vi "Main.vi"(11 "Error in":errorcluster) -> (15 "Error out":errorcluster)   [LabVIEW 2020, in "PSRR Monitor.lvlib"]
uses:
  PSRR Monitor.lvlib
  Typedefs/Queue operations.ctl
  Typedefs/Data Cluster.ctl
  Typedefs/Variant cluster.ctl
  Typedefs/User LV2 operations.ctl
  Typedefs/User LV2 data.ctl
  <vilib>/Utility/config.llb/Read Key (I32).vi
  <vilib>/Utility/config.llb/Read Key (Boolean).vi
  SubVI/Error log.vi
  <vilib>/Utility/config.llb/Write Key (I32).vi
  <vilib>/Utility/config.llb/Write Key (Boolean).vi
  <vilib>/Utility/config.llb/NI_LVConfig.lvlib
panel:
  out "Obtained PSRR":i32(graph)
  in  "Error Log":bool
  in  "Exit":bool
  out "Description":string
  out "Time":string
  out "Type":string
  out "Error Code":i32
  out "Last Read PSRR (dB)":i32
  in  "Wait Time(sec)":i32 min=2 step=1
  out "Error?":bool
  # "PSRR MONITOR"
  # "Power Supply Rejection Ratio"
  # "Last Error Details"
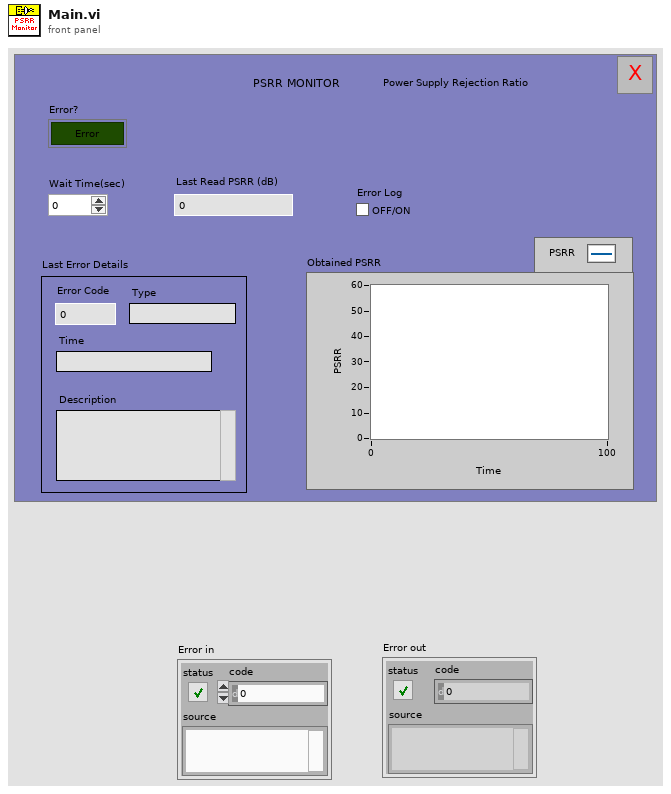
[diagram p1: front panel]
types:
  T1 = typedef "User LV2 operations.ctl" = enum16{"Destroy", "Get ref", "Generate", "Create"}
  T2 = typedef "PSRR Monitor.lvlib/Variant cluster.ctl" = cluster{"State":string, "Data":variant}
  T3 = typedef "PSRR Monitor.lvlib/Queue operations.ctl" = enum16{"Create", "Enqueue", "Enstack", "Dequeue", "Flush", "Release "}
  T4 = typedef "PSRR Monitor.lvlib/Data Cluster.ctl" = cluster{"Error?":bool, "Exit":bool, "Error log":bool, "Type":string, "Time":string, "Description":string, "Wait Time":i32, "Last Read PSRR":i32, "Error code":i32, "Obtained PSRR":i32, "Start/Stop Timer":bool, "Start time":dbl, "Path":path, "Passive count":dbl, "Other error count":dbl}
  T5 = typedef "User LV2 data.ctl" = cluster{"Exit":bool}
  T6 = typedef "NI_LVConfig.lvlib/Config Data RefNum.ctl" = refnum<k1>
  T7 = enum32{"Bad", "Idle", "Run top level", "Running"}
  T8 = typedef "PSRR Monitor.lvlib/Error Details.ctl" = cluster{"Error Code":i32, "Error Type":string, "Time":string, "Description":string, "PSRR":i32}
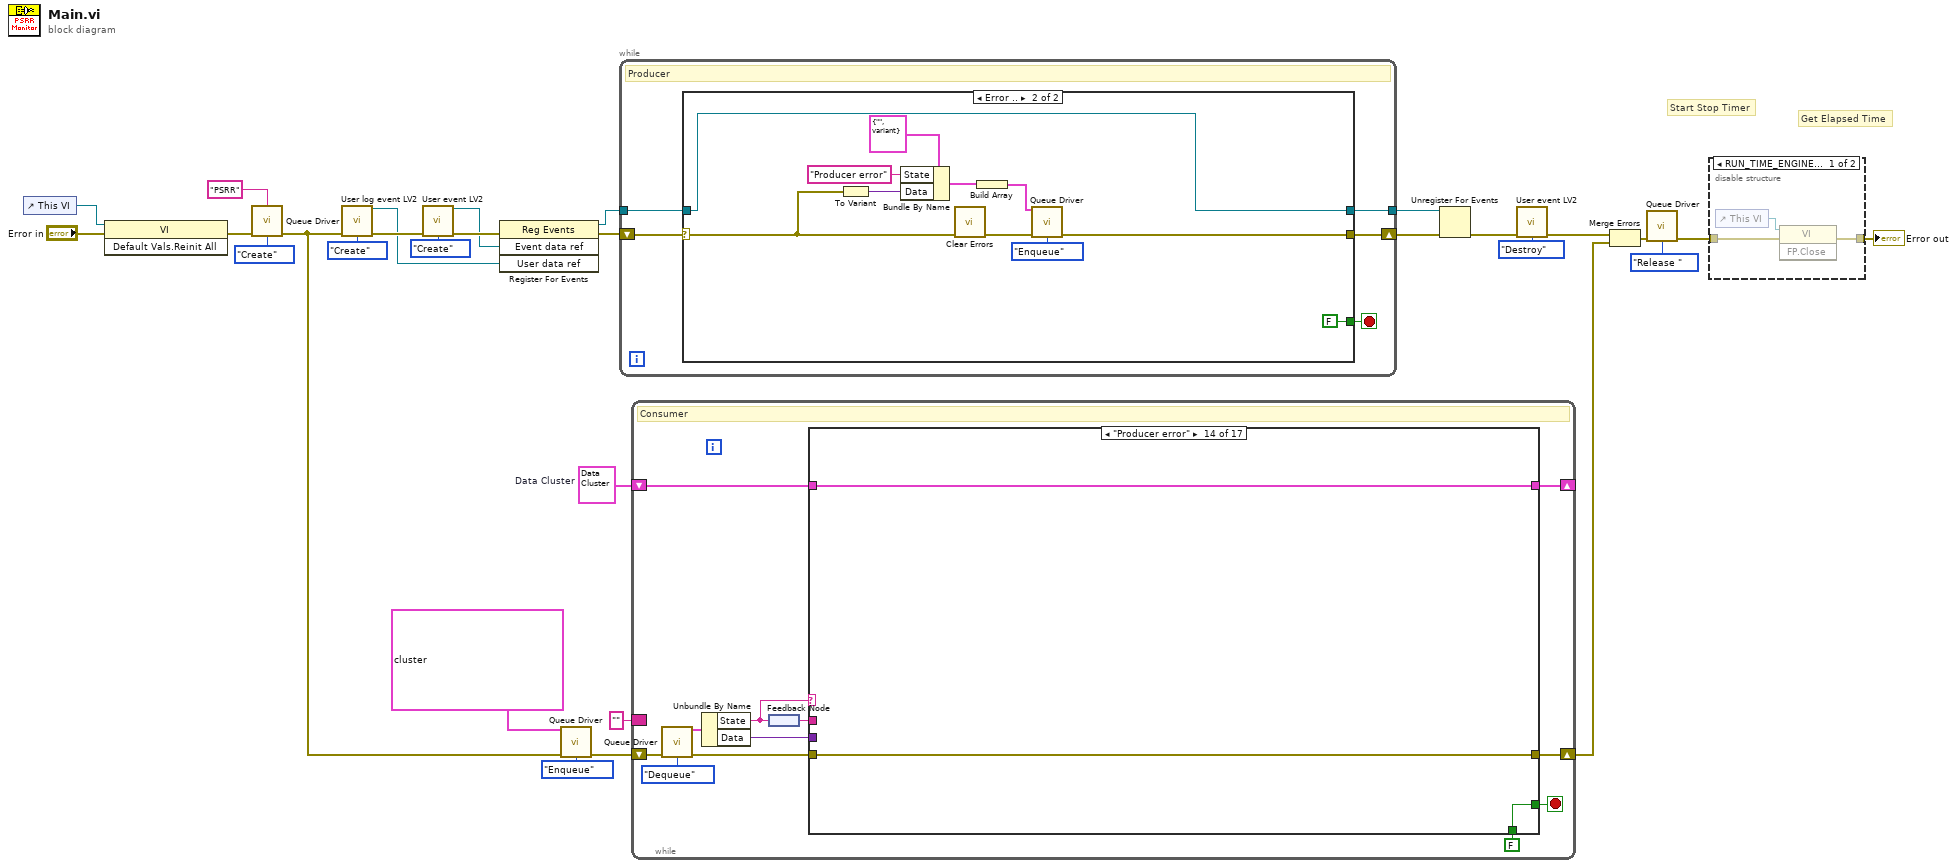
[diagram p0: block diagram]
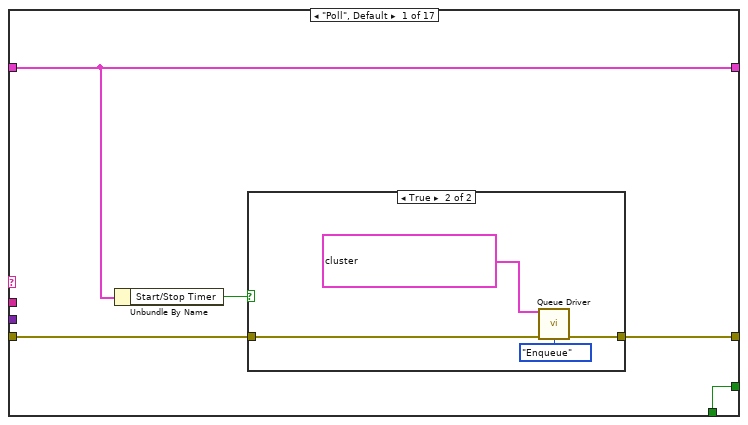
[diagram p3: hidden frame]
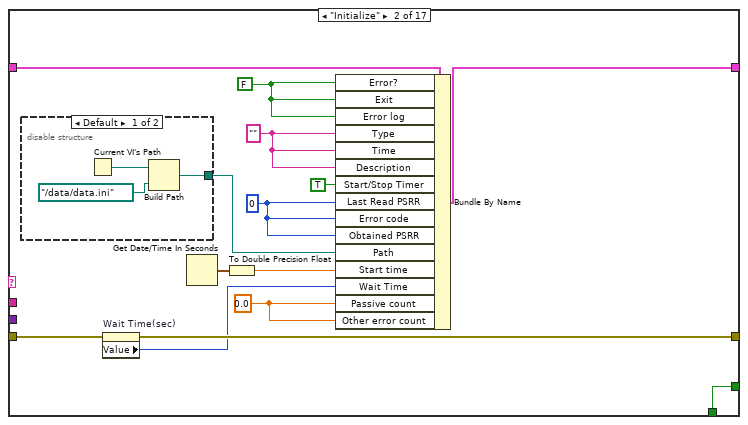
[diagram p5: hidden frame]
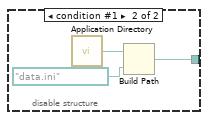
[diagram p6: hidden frame]
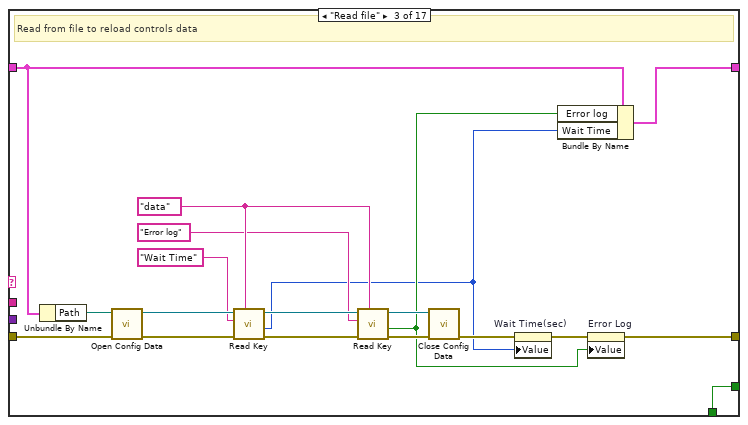
[diagram p7: hidden frame]
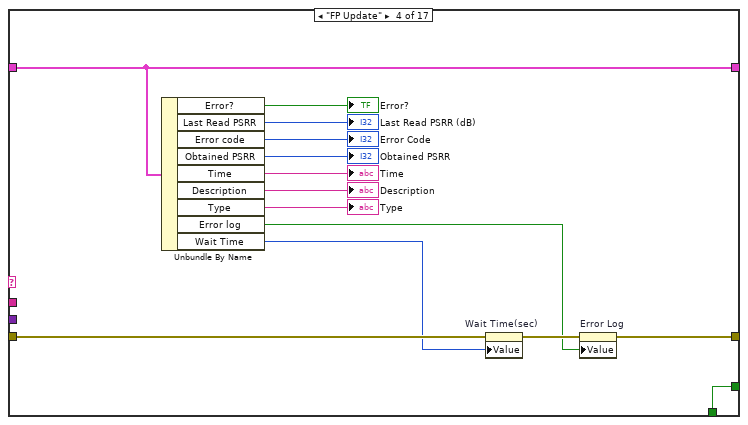
[diagram p8: hidden frame]
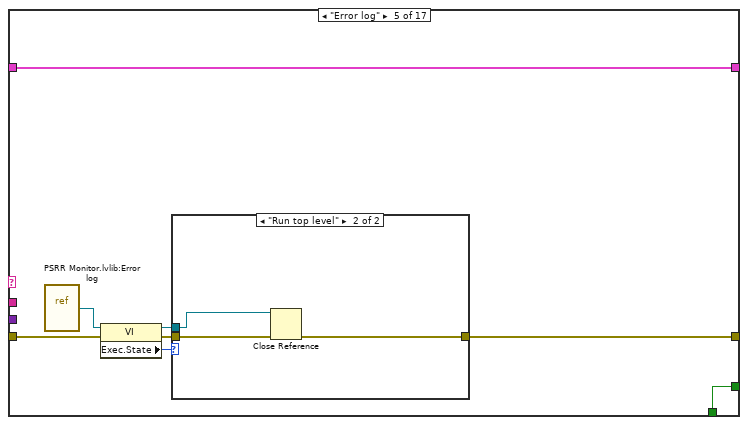
[diagram p9: hidden frame]
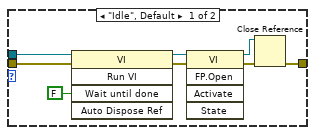
[diagram p10: hidden frame]
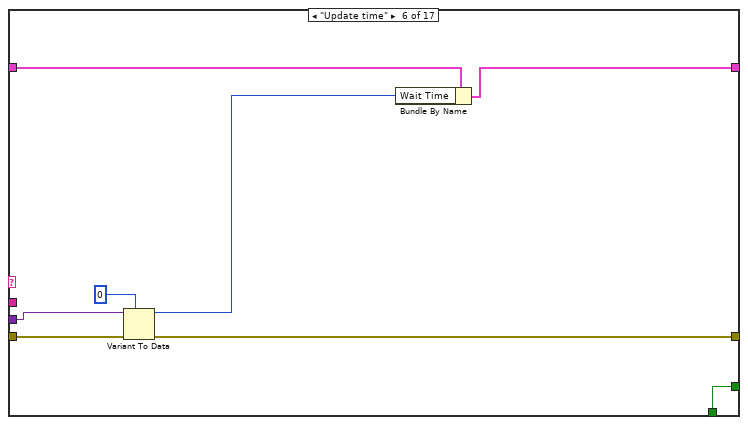
[diagram p11: hidden frame]
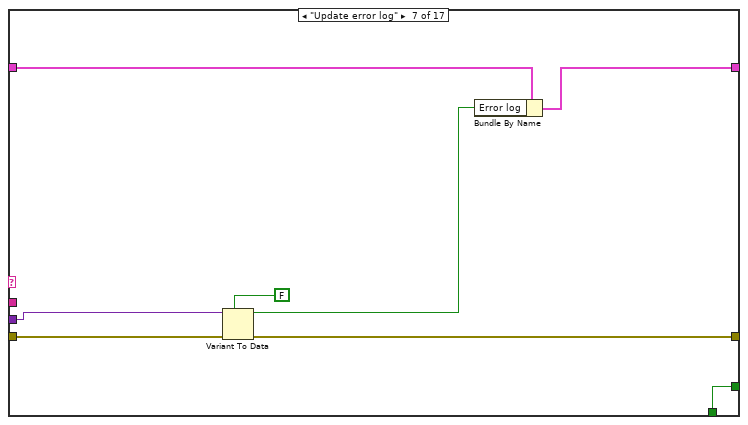
[diagram p12: hidden frame]
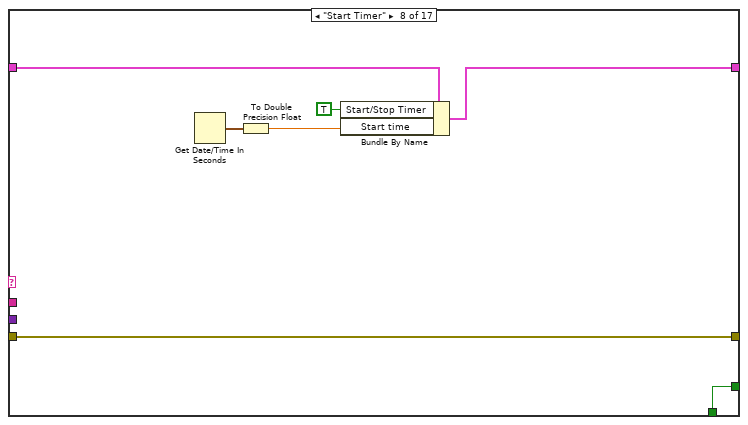
[diagram p13: hidden frame]
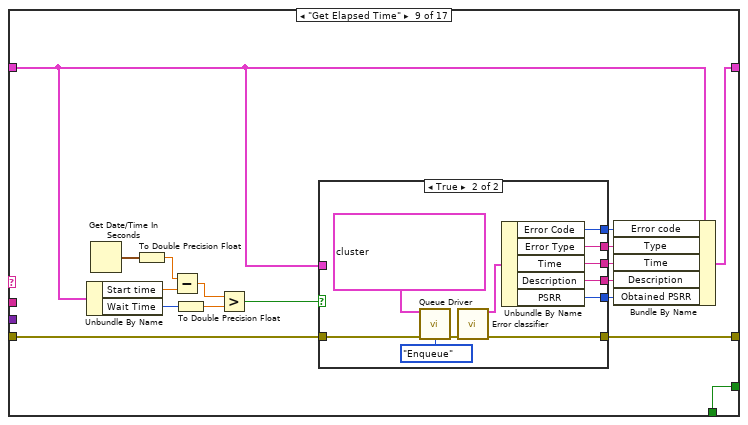
[diagram p14: hidden frame]
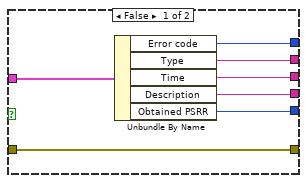
[diagram p15: hidden frame]
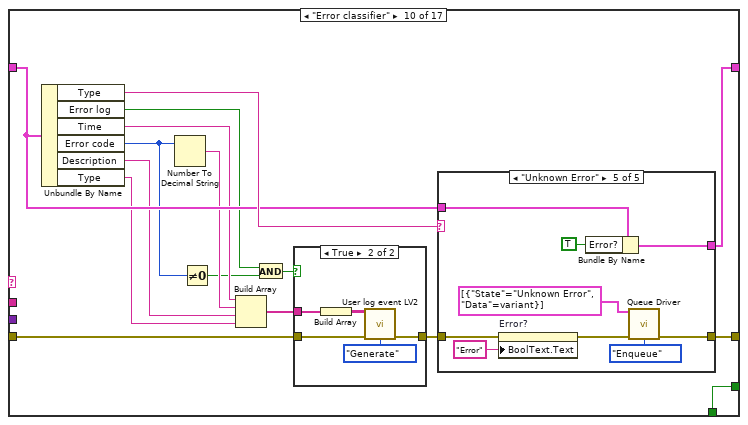
[diagram p16: hidden frame]
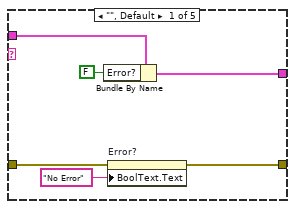
[diagram p18: hidden frame]
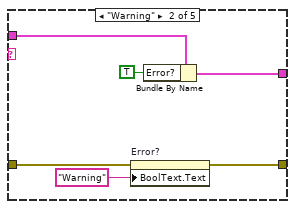
[diagram p19: hidden frame]
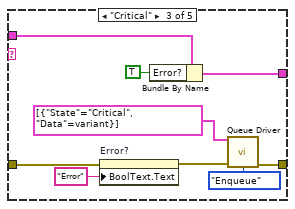
[diagram p20: hidden frame]
diagram:
  w24 = T4 {"Error?"=FALSE, "Exit"=FALSE, "Error log"=FALSE, "Type"="", "Time"="", "Description"="", "Wait Time"=0, "Last Read PSRR"=0, "Error code"=0, "Obtained PSRR"=0, "Start/Stop Timer"=FALSE, "Start time"=0.0, "Path"=path "", "Passive count"=0.0, "Other error count"=0.0}  # Data Cluster
  # "Get Elapsed Time"
  # "Start Stop Timer"
  n1 = control-ref of="This VI"() -> (w17:refnum<vi>)
  n2 = invoke class="VI" method="Default Vals.Reinit All"(reference=w17, error in="Error in") -> (error out=w15:errorcluster)  [unwired: 1 in, 2 out]
  n3 = call "Queue Driver.vi"("Name"="PSRR", "Error in"=w15, "Queue Operations"=Queue_operations."Create") -> ("Error out"=w3:errorcluster)  [unwired: 11 in, 1 out]
  n4 = call "User log event LV2.vi"("Error in"=w3, "Operation"=User_LV2_operations."Create") -> ("User data ref"=w1:refnum<user-event>, "Error out"=w2:errorcluster)  [unwired: 12 in]
  n5 = call "User event LV2.vi"("Error in"=w2, "Operation"=User_LV2_operations."Create") -> ("Event data ref"=w11:refnum<user-event>, "Error out"=w13:errorcluster)  [unwired: 12 in]
  n6 = register-events(error in=w13, w11, w1) -> (reference out=w10:refnum<event-registration>, error out=w12:errorcluster)  [unwired: 1 in]
  n7 = call "Queue Driver.vi"("State and data"=T2[] [{"State"="Initialize", "Data"=variant}, {"State"="Read file", "Data"=variant}, {"State"="FP Update", "Data"=variant}, {"State"="Error log", "Data"=variant}], "Error in"=w3, "Queue Operations"=Queue_operations."Enqueue") -> ("Error out"=w26:errorcluster)  [unwired: 11 in, 1 out]
  n8 = while {
    shift-right: [w33] -> w9
    shift-left: w12 -> [w34]
    tunnel: w10 -> [w31]
    tunnel: [w30] -> w8
    stop <- w32 stop-if-true
    # "Producer"
    n9 = case shown="Error .." w34 {
      selector: w34 -> [w38 w83]
      tunnel: [w39 w89] -> w33
      tunnel: [w37 FALSE ("Discard?")] -> w32
      tunnel: w31 -> [w36 w81]
      tunnel: [w35 w81] -> w30
      frame No Error {
        n10 = event shown="[5] Panel Close?" {
          selector: w36 -> [_ _ _ _ _ _]
          dyn-events: [_ _ _ _ _ _] -> w35
          timeout: 50 -> [_ _ _ _ _ _]
          tunnel: [w42 w49 w54 w64 w65 w73] -> w39
          tunnel: w38 -> [w42 w50 w55 w64 w70 w78]
          tunnel: [FALSE ("Discard?") FALSE ("Discard?") FALSE ("Discard?") TRUE ("Discard?") TRUE ("Discard?") w80] -> w37
          event Timeout {
            n11 = event-data() -> ()  [unwired: 1 in, 1 out]
          }
          event "Wait Time(sec)": Value Change {
            n12 = event-data() -> ("NewVal"=w48:i32)  [unwired: 1 in]
            n13 = To Variant(anything=w48) -> (Variant=w46:variant)
            n14 = Bundle By Name(cluster=T2 {"State"="", "Data"=variant} ("Dequeued output"), "State"="Update time", "Data"=w46) -> (w44:T2)
            n15 = Build Array(w44) -> (w43:T2[])
            n16 = call "Queue Driver.vi"("State and data"=w43, "Error in"=w50, "Queue Operations"=Queue_operations."Enqueue") -> ("Error out"=w49:errorcluster)  [unwired: 11 in, 1 out]
          }
          event "Error Log": Value Change {
            n17 = event-data() -> ("NewVal"=w58:bool)  [unwired: 1 in]
            n18 = To Variant(anything=w58) -> (Variant=w60:variant)
            n19 = Bundle By Name(cluster=T2 {"State"="", "Data"=variant} ("Dequeued output"), "State"="Update error log", "Data"=w60) -> (w57:T2)
            n20 = Build Array(w57) -> (w53:T2[])
            n21 = call "Queue Driver.vi"("State and data"=w53, "Error in"=w55, "Queue Operations"=Queue_operations."Enqueue") -> ("Error out"=w54:errorcluster)  [unwired: 11 in, 1 out]
          }
          event User Event {
            n22 = event-data() -> ()  [unwired: 1 in, 1 out]
          }
          event "Exit": Value Change {
            n23 = event-data() -> ()  [unwired: 1 in, 1 out]
            n24 = call "Queue Driver.vi"("State and data"=T2[] [{"State"="Write file", "Data"=variant}, {"State"="Exit", "Data"=variant}], "Error in"=w70, "Queue Operations"=Queue_operations."Enqueue") -> ("Error out"=w66:errorcluster)  [unwired: 11 in, 1 out]
            n25 = call "User event LV2.vi"("Event data"=T5 {"Exit"=TRUE}, "Error in"=w66, "Operation"=User_LV2_operations."Generate") -> ("Error out"=w65:errorcluster)  [unwired: 11 in, 1 out]
          }
          event Panel Close? {
            w80 = TRUE ("Discard?")
            n26 = event-data() -> ()  [unwired: 1 in, 1 out]
            n27 = call "Queue Driver.vi"("State and data"=T2[] [{"State"="Write file", "Data"=variant}, {"State"="Exit", "Data"=variant}], "Error in"=w78, "Queue Operations"=Queue_operations."Enqueue") -> ("Error out"=w74:errorcluster)  [unwired: 11 in, 1 out]
            n28 = call "User event LV2.vi"("Event data"=T5 {"Exit"=TRUE}, "Error in"=w74, "Operation"=User_LV2_operations."Generate") -> ("Error out"=w73:errorcluster)  [unwired: 11 in, 1 out]
            n29 = event-data("Discard?"=w80) -> ()  [unwired: 1 in, 1 out]
          }
        }
      }
      frame Error {
        n30 = To Variant(anything=w83) -> (Variant=w82:variant)
        n31 = Bundle By Name(cluster=T2 {"State"="", "Data"=variant} ("Dequeued output"), "State"="Producer error", "Data"=w82) -> (w86:T2)
        n32 = call <vilib>:"Clear Errors.vi"("error in (no error)"=w83) -> ("error out"=w88:errorcluster)  [unwired: 5 in, 1 out]
        n33 = Build Array(w86) -> (w85:T2[])
        n34 = call "Queue Driver.vi"("State and data"=w85, "Error in"=w88, "Queue Operations"=Queue_operations."Enqueue") -> ("Error out"=w89:errorcluster)  [unwired: 11 in, 1 out]
      }
    }
  }
  n35 = while {
    shift-right: [w95] -> w23
    shift-left: w26 -> [w102]
    border: "" ("State") -> [_]
    shift-right: [w96] -> _
    shift-left: w24 -> [w97]
    stop <- w94 stop-if-true
    # "Consumer"
    n36 = call "Queue Driver.vi"("Error in"=w102, "Queue Operations"=Queue_operations."Dequeue") -> ("Dequeued output"=w101:T2, "Error out"=w99:errorcluster)  [unwired: 12 in]
    n37 = Unbundle By Name(w101) -> ("State"=w92:string, "Data"=w100:variant)
    n38 = feedback-in #1(w92) -> ()
    n39 = feedback #1() -> (w98:string)
    n40 = case shown="\"Producer error\"" w92 {
      tunnel: w100 -> [_ _ _ _ _ w187 w197 _ _ _ _ _ _ _ _ _ _]
      tunnel: w99 -> [w107 w116 w151 w157 w171 w190 w199 w208 w221 w253 w314 w337 w358 w375 w378 w395 w398]
      tunnel: w97 -> [w105 w127 w137 w165 w174 w192 w196 w203 w212 w256 w307 w335 w365 w376 w379 w392 w401]
      tunnel: [w105 w123 w136 w165 w174 w191 w195 w202 w218 w255 w306 w333 w365 w376 w379 w392 w401] -> w96
      tunnel: [w106 w115 w138 w155 w167 w189 w198 w208 w220 w257 w313 w336 w359 w375 w378 w393 w397] -> w95
      tunnel: [w108 w122 w152 w166 w173 w193 w201 w207 w209 w259 w315 w340 w364 w374 w377 w396 TRUE] -> w94
      tunnel: FALSE -> [w108 w122 w152 w166 w173 w193 w201 w207 w209 w259 w315 w340 w364 w374 w377 w396 _]
      tunnel: w98 -> [_ _ _ _ _ _ _ _ _ _ _ _ _ _ _ _ _]
      frame "Poll", Default {
        n41 = Unbundle By Name(w105) -> ("Start/Stop Timer"=w104:bool)
        n42 = case shown="True" w104 {
          tunnel: w107 -> [w109 w112]
          tunnel: [w109 w111] -> w106
          frame False {
          }
          frame True {
            n43 = call "Queue Driver.vi"("State and data"=T2[] [{"State"="Get Elapsed Time", "Data"=variant}, {"State"="FP Update", "Data"=variant}], "Error in"=w112, "Queue Operations"=Queue_operations."Enqueue") -> ("Error out"=w111:errorcluster)  [unwired: 11 in, 1 out]
          }
        }
      }
      frame "Initialize" {
        w118 = 0.0 ("Passive count")
        w124 = "" ("Type")
        w125 = FALSE ("Error?")
        w126 = 0 ("Last Read PSRR")
        n44 = disable-structure shown="Default" {
          disable-tunnel: [w128 w132] -> w119
          frame condition #0 (active) {
            n45 = Current VI's Path() -> (path=w130:path)
            n46 = Build Path(base path=w130, name or relative path=path "../data/data.ini") -> (appended path=w128:path)
          }
          frame condition #1 {
            n47 = call <vilib>:"Application Directory.vi"() -> ("Application Directory"=w131:path)
            n48 = Build Path(base path=w131, name or relative path=path "data.ini") -> (appended path=w132:path)
          }
        }
        n49 = property on="Wait Time(sec)" class="DigNum (strict)"(error in=w116) -> (error out=w115:errorcluster, "Value"=w114:i32)  [unwired: 1 in, 1 out]
        n50 = Get Date/Time In Seconds() -> (seconds since 1Jan1904=w121:timestamp)
        n51 = To Double Precision Float(number=w121) -> (double precision float=w120:dbl)
        n52 = Bundle By Name(cluster=w127, "Error?"=w125, "Exit"=w125, "Error log"=w125, "Type"=w124, "Time"=w124, "Description"=w124, "Start/Stop Timer"=TRUE, "Last Read PSRR"=w126, "Error code"=w126, "Obtained PSRR"=w126, "Path"=w119, "Start time"=w120, "Wait Time"=w114, "Passive count"=w118, "Other error count"=w118) -> (w123:T4)
      }
      frame "Read file" {
        w143 = "data" ("section")
        # "Read from file to reload controls data"
        n53 = Unbundle By Name(w137) -> ("Path"=w144:path)
        n54 = call <vilib>:"Open Config Data.vi"("error in (no error)"=w151, "configuration file path"=w144) -> ("error out"=w150:errorcluster, "refnum"=w147:T6)  [unwired: 7 in, 1 out]
        n55 = call-poly <vilib>:"Read Key.vi"("section"=w143, "error in (no error)"=w150, "key"="Wait Time", "refnum"=w147) -> ("error out"=w149:errorcluster, "value"=w134:i32, "refnum out"=w146:T6)  [unwired: 4 in, 1 out]
        n56 = call-poly <vilib>:"Read Key.vi"("section"=w143, "error in (no error)"=w149, "key"="Error log", "refnum"=w146) -> ("error out"=w148:errorcluster, "value"=w135:bool, "refnum out"=w145:T6)  [unwired: 4 in, 1 out]
        n57 = call <vilib>:"Close Config Data.vi"("error in (no error)"=w148, "refnum"=w145) -> ("error out"=w140:errorcluster)  [unwired: 8 in, 1 out]
        n58 = property on="Wait Time(sec)" class="DigNum (strict)"(error in=w140, "Value"=w134) -> (error out=w139:errorcluster)  [unwired: 1 in, 1 out]
        n59 = Bundle By Name(cluster=w137, "Error log"=w135, "Wait Time"=w134) -> (w136:T4)
        n60 = property on="Error Log" class="Bool (strict)"(error in=w139, "Value"=w135) -> (error out=w138:errorcluster)  [unwired: 1 in, 1 out]
      }
      frame "FP Update" {
        n61 = Unbundle By Name(w165) -> ("Error?"=→"Error?":bool, "Last Read PSRR"=→"Last Read PSRR (dB)":i32, "Error code"=→"Error Code":i32, "Obtained PSRR"=→"Obtained PSRR":i32, "Time"=→"Time":string, "Description"=→"Description":string, "Type"=→"Type":string, "Error log"=w153:bool, "Wait Time"=w154:i32)
        n62 = property on="Wait Time(sec)" class="DigNum (strict)"(error in=w157, "Value"=w154) -> (error out=w156:errorcluster)  [unwired: 1 in, 1 out]
        n63 = property on="Error Log" class="Bool (strict)"(error in=w156, "Value"=w153) -> (error out=w155:errorcluster)  [unwired: 1 in, 1 out]
      }
      frame "Error log" {
        n64 = vi-ref "PSRR Monitor.lvlib:Error log.vi"() -> (w172:refnum<vi>)
        n65 = property class="VI"(reference=w172, error in=w171) -> (reference out=w168:refnum<vi>, error out=w169:errorcluster, "Exec.State"=w170:T7)
        n66 = case shown="\"Run top level\"" w170 {
          tunnel: w169 -> [w182 w184]
          tunnel: w168 -> [w180 w185]
          tunnel: [w179 w183] -> w167
          frame "Idle", Default {
            n67 = invoke class="VI" method="Run VI"(reference=w180, error in=w182, "Wait until done"=FALSE ("Wait Until Done")) -> (reference out=w176:refnum<vi>, error out=w178:errorcluster)  [unwired: 2 in, 3 out]
            n68 = invoke class="VI" method="FP.Open"(reference=w176, error in=w178) -> (reference out=w175:refnum<vi>, error out=w177:errorcluster)  [unwired: 3 in, 3 out]
            n69 = Close Reference(reference=w175, error in (no error)=w177) -> (error out=w179:errorcluster)
          }
          frame "Run top level" {
            n70 = Close Reference(reference=w185, error in (no error)=w184) -> (error out=w183:errorcluster)
          }
        }
      }
      frame "Update time" {
        n71 = Variant To Data(error in=w190, type=0 ("NewVal"), Variant=w187) -> (data=w188:i32, error out=w189:errorcluster)
        n72 = Bundle By Name(cluster=w192, "Wait Time"=w188) -> (w191:T4)
      }
      frame "Update error log" {
        n73 = Variant To Data(error in=w199, type=FALSE, Variant=w197) -> (data=w194:bool, error out=w198:errorcluster)
        n74 = Bundle By Name(cluster=w196, "Error log"=w194) -> (w195:T4)
      }
      frame "Start Timer" {
        n75 = Get Date/Time In Seconds() -> (seconds since 1Jan1904=w205:timestamp)
        n76 = To Double Precision Float(number=w205) -> (double precision float=w206:dbl)
        n77 = Bundle By Name(cluster=w203, "Start/Stop Timer"=TRUE, "Start time"=w206) -> (w202:T4)
      }
      frame "Get Elapsed Time" {
        n78 = Unbundle By Name(w212) -> ("Start time"=w224:dbl, "Wait Time"=w222:i32)
        n79 = Get Date/Time In Seconds() -> (seconds since 1Jan1904=w225:timestamp)
        n80 = To Double Precision Float(number=w225) -> (double precision float=w223:dbl)
        n81 = Subtract(x=w223, y=w224) -> (x-y=w210:dbl)
        n82 = To Double Precision Float(number=w222) -> (double precision float=w211:dbl)
        n83 = Greater?(x=w210, y=w211) -> (0:w219:bool)
        n84 = case shown="True" w219 {
          tunnel: w221 -> [w232 w235]
          tunnel: [w232 w243] -> w220
          tunnel: [w230 w241] -> w217
          tunnel: [w229 w240] -> w216
          tunnel: [w228 w239] -> w215
          tunnel: [w227 w238] -> w214
          tunnel: [w226 w237] -> w213
          tunnel: w212 -> [w231 _]
          frame False {
            n85 = Unbundle By Name(w231) -> ("Error code"=w230:i32, "Type"=w229:string, "Time"=w228:string, "Description"=w227:string, "Obtained PSRR"=w226:i32)
          }
          frame True {
            n86 = call "Queue Driver.vi"("State and data"=T2[] [{"State"="FP Update", "Data"=variant}, {"State"="Error classifier", "Data"=variant}, {"State"="Start Timer", "Data"=variant}], "Error in"=w235, "Queue Operations"=Queue_operations."Enqueue") -> ("Error out"=w234:errorcluster)  [unwired: 11 in, 1 out]
            n87 = call "Error classifier.vi"("Error in"=w234) -> ("Classified Ouput Error"=w242:T8, "Error out"=w243:errorcluster)  [unwired: 13 in]
            n88 = Unbundle By Name(w242) -> ("Error Code"=w241:i32, "Error Type"=w240:string, "Time"=w239:string, "Description"=w238:string, "PSRR"=w237:i32)
          }
        }
        n89 = Bundle By Name(cluster=w212, "Error code"=w217, "Type"=w216, "Time"=w215, "Description"=w214, "Obtained PSRR"=w213) -> (w218:T4)
      }
      frame "Error classifier" {
        n90 = Unbundle By Name(w256) -> ("Type"=w258:string, "Error log"=w244:bool, "Time"=w250:string, "Error code"=w247:i32, "Description"=w251:string, "Type"=w249:string)
        n91 = Number To Decimal String(number=w247) -> (decimal integer string=w252:string)  [unwired: 1 in]
        n92 = Not Equal To 0?(x=w247) -> (x != 0?=w245:bool)
        n93 = Build Array(w250, w252, w251, w249) -> (w248:string[])
        n94 = And(x=w244, y=w245) -> (x .and. y?=w246:bool)
        n95 = case shown="True" w246 {
          tunnel: [w260 w263] -> w254
          tunnel: w253 -> [w260 w264]
          tunnel: w248 -> [_ w262]
          frame False {
          }
          frame True {
            n96 = Build Array(w262) -> (w261:string[][])
            n97 = call "User log event LV2.vi"("User Data"=w261, "Error in"=w264, "Operation"=User_LV2_operations."Generate") -> ("Error out"=w263:errorcluster)  [unwired: 11 in, 1 out]
          }
        }
        n98 = case shown="\"Unknown Error\"" w258 {
          tunnel: w254 -> [w271 w274 w279 w288 w297]
          tunnel: [w270 w273 w285 w294 w303] -> w257
          tunnel: w256 -> [w268 w277 w283 w291 w301]
          tunnel: [w267 w276 w282 w292 w300] -> w255
          frame "", Default {
            n99 = Bundle By Name(cluster=w268, "Error?"=FALSE) -> (w267:T4)
            n100 = property on="Error?" class="Bool (strict)"(error in=w271, "BoolText.Text"="No Error" ("Boolean Text.Text")) -> (error out=w270:errorcluster)  [unwired: 1 in, 1 out]
          }
          frame "Warning" {
            n101 = property on="Error?" class="Bool (strict)"(error in=w274, "BoolText.Text"="Warning" ("Boolean Text.Text")) -> (error out=w273:errorcluster)  [unwired: 1 in, 1 out]
            n102 = Bundle By Name(cluster=w277, "Error?"=TRUE) -> (w276:T4)
          }
          frame "Critical" {
            n103 = property on="Error?" class="Bool (strict)"(error in=w279, "BoolText.Text"="Error" ("Boolean Text.Text")) -> (error out=w278:errorcluster)  [unwired: 1 in, 1 out]
            n104 = Bundle By Name(cluster=w283, "Error?"=TRUE) -> (w282:T4)
            n105 = call "Queue Driver.vi"("State and data"=T2[] [{"State"="Critical", "Data"=variant}], "Error in"=w278, "Queue Operations"=Queue_operations."Enqueue") -> ("Error out"=w285:errorcluster)  [unwired: 11 in, 1 out]
          }
          frame "Passive" {
            n106 = property on="Error?" class="Bool (strict)"(error in=w288, "BoolText.Text"="Error" ("Boolean Text.Text")) -> (error out=w287:errorcluster)  [unwired: 1 in, 1 out]
            n107 = Bundle By Name(cluster=w291, "Error?"=TRUE) -> (w292:T4)
            n108 = call "Queue Driver.vi"("State and data"=T2[] [{"State"="Passive", "Data"=variant}], "Error in"=w287, "Queue Operations"=Queue_operations."Enqueue") -> ("Error out"=w294:errorcluster)  [unwired: 11 in, 1 out]
          }
          frame "Unknown Error" {
            n109 = property on="Error?" class="Bool (strict)"(error in=w297, "BoolText.Text"="Error" ("Boolean Text.Text")) -> (error out=w296:errorcluster)  [unwired: 1 in, 1 out]
            n110 = Bundle By Name(cluster=w301, "Error?"=TRUE) -> (w300:T4)
            n111 = call "Queue Driver.vi"("State and data"=T2[] [{"State"="Unknown Error", "Data"=variant}], "Error in"=w296, "Queue Operations"=Queue_operations."Enqueue") -> ("Error out"=w303:errorcluster)  [unwired: 11 in, 1 out]
          }
        }
      }
      frame "Unknown Error" {
        # "Unknown error information for user"
        n112 = Unbundle By Name(w307) -> ("Description"=w309:string, "Other error count"=w312:dbl, "Other error count"=w305:dbl)
        n113 = Greater Or Equal?(x=w312, y=3.0) -> (x >= y?=w310:bool)
        n114 = case shown="True" w310 {
          tunnel: w314 -> [w320 w332]
          tunnel: [w320 w332] -> w313
          tunnel: w309 -> [_ w331]
          tunnel: "Occurred with code at  " ("string") -> [_ w330]
          tunnel: w307 -> [w319 w326]
          tunnel: [w318 w325] -> w306
          tunnel: w305 -> [w316 _]
          frame False {
            n115 = Increment(x=w316) -> (x+1=w317:dbl)
            n116 = Bundle By Name(cluster=w319, "Other error count"=w317) -> (w318:T4)
          }
          frame True {
            n117 = Concatenate Strings(w330, w331) -> (w329:string)
            n118 = Two Button Dialog(message=w329, 1:"Acknowledge next" ("F button name (\"Cancel\")"), 2:"Continue" ("T button name (\"OK\")")) -> (T button?=w324:bool)
            n119 = Select(t=0.0, s=w324, f=3.0) -> (s? t:f=w321:dbl)
            n120 = Bundle By Name(cluster=w326, "Other error count"=w321) -> (w325:T4)
          }
        }
      }
      frame "Passive" {
        # "Passive information and acknowledgement from the user"
        n121 = Unbundle By Name(w335) -> ("Passive count"=w334:dbl)
        n122 = Greater Or Equal?(x=w334, y=3.0) -> (x >= y?=w338:bool)
        n123 = case shown="False" w338 {
          tunnel: w337 -> [w345 w355]
          tunnel: [w345 w355] -> w336
          tunnel: w335 -> [w344 w351]
          tunnel: w334 -> [w342 _]
          tunnel: [w341 w350] -> w333
          frame False {
            # "Continue"
            n124 = Increment(x=w342) -> (x+1=w343:dbl)
            n125 = Bundle By Name(cluster=w344, "Passive count"=w343) -> (w341:T4)
          }
          frame True {
            # "Pop up for user if error occurred thrice"
            n126 = Two Button Dialog(message="Passive error has occurred", 1:"Acknowledge next" ("F button name (\"Cancel\")"), 2:"Continue" ("T button name (\"OK\")")) -> (T button?=w348:bool)
            n127 = Select(t=0.0, s=w348, f=2.0) -> (s? t:f=w349:dbl)
            n128 = Bundle By Name(cluster=w351, "Passive count"=w349) -> (w350:T4)
          }
        }
      }
      frame "Critical" {
        # "Critical information for user"
        n129 = property on="Obtained PSRR" class="WFChart (strict)"(error in=w358, "History Data"=i32[] []) -> (error out=w357:errorcluster)  [unwired: 1 in, 1 out]
        n130 = Two Button Dialog(message="Critical Error has occurred", 1:"Exit" ("F button name (\"Cancel\")"), 2:"Continue" ("T button name (\"OK\")")) -> (T button?=w360:bool)
        n131 = case shown="True" w360 {
          tunnel: w357 -> [w368 w373]
          tunnel: [w371 w373] -> w359
          frame False {
            n132 = call "User event LV2.vi"("Event data"=T5 {"Exit"=TRUE}, "Error in"=w368, "Operation"=User_LV2_operations."Generate") -> ("Error out"=w367:errorcluster)  [unwired: 11 in, 1 out]
            n133 = call "Queue Driver.vi"("State and data"=T2[] [{"State"="Write file", "Data"=variant}, {"State"="Exit", "Data"=variant}], "Error in"=w367, "Queue Operations"=Queue_operations."Enqueue") -> ("Error out"=w371:errorcluster)  [unwired: 11 in, 1 out]
          }
          frame True {
          }
        }
      }
      frame "Producer error" {
      }
      frame "Error" {
      }
      frame "Write file" {
        w387 = "data" ("section")
        n134 = Unbundle By Name(w392) -> ("Error log"=w380:bool, "Wait Time"=w381:i32, "Path"=w391:path)
        n135 = call <vilib>:"Open Config Data.vi"("error in (no error)"=w395, "create file if necessary (T)"=FALSE, "configuration file path"=w391) -> ("error out"=w394:errorcluster, "refnum"=w390:T6)  [unwired: 6 in, 1 out]
        n136 = call-poly <vilib>:"Write Key.vi"("section"=w387, "error in (no error)"=w394, "value"=w381, "key"="Wait Time", "refnum"=w390) -> ("error out"=w389:errorcluster, "refnum out"=w386:T6)  [unwired: 4 in, 1 out]
        n137 = call-poly <vilib>:"Write Key.vi"("section"=w387, "error in (no error)"=w389, "value"=w380, "key"="Error log", "refnum"=w386) -> ("error out"=w388:errorcluster, "refnum out"=w385:T6)  [unwired: 4 in, 1 out]
        n138 = call <vilib>:"Close Config Data.vi"("error in (no error)"=w388, "refnum"=w385) -> ("error out"=w393:errorcluster)  [unwired: 8 in, 1 out]
      }
      frame "Exit" {
        # "Release and terminate loop"
        n139 = call "Queue Driver.vi"("Error in"=w398, "Queue Operations"=Queue_operations."Flush") -> ("Error out"=w397:errorcluster)  [unwired: 12 in, 1 out]
      }
    }
  }
  n140 = Unregister For Events(event registration refnum=w8, error in=w9) -> (error out=w6:errorcluster)
  n141 = call "User event LV2.vi"("Error in"=w6, "Operation"=User_LV2_operations."Destroy") -> ("Error out"=w5:errorcluster)  [unwired: 12 in, 1 out]
  n142 = Merge Errors(w5, w23) -> (w21:errorcluster)
  n143 = call "Queue Driver.vi"("Error in"=w21, "Queue Operations"=Queue_operations."Release ") -> ("Error out"=w20:errorcluster)  [unwired: 12 in, 1 out]
  n144 = disable-structure shown="RUN_TIME_ENGINE==True" {
    disable-tunnel: w20 -> [w404 w405]
    disable-tunnel: [w402 w405] -> w19
    frame condition #0 {
      n145 = control-ref of="This VI"() -> (w403:refnum<vi>)
      n146 = invoke class="VI" method="FP.Close"(reference=w403, error in=w404) -> (error out=w402:errorcluster)  [unwired: 1 in, 2 out]
    }
    frame condition #1 (active) {
    }
  }
  "Error out" <- w19
